vi "AI Read with state .vi"(0 "taskID in":u32 format="%x", 1 "conditional retrieval (off)":T2={"mode (off)"=enum."off", "channel index (0)"=0, "slope (rising)"=enum."rising", "level (0.0)"=0.0, "hysteresis (0.0)"=0.0, "skip count (0)"=0, "offset (0)"=0} {"hysteresis (0.0)" format="%0.2f"; "level (0.0)" format="%0.2f"}, 5 "number of scans to read (-1:all)":i32=-1, 7 "time limit in sec (-1:auto calculate)":sgl=-1.0 format="%0.2f", 11 "error in (no error)":errorcluster, 12 "read/search position (from mark)":T3={"position (rel. to mark:1)"=enum."relative to read mark", "read offset (0)"=0}) -> (2 "scan backlog":u32, 3 "number read":i32, 4 "taskID out":u32 format="%x", 6 "scaled data":sgl[][](array[numeric]) format="%0.6f", 10 "retrieval complete":bool, 14 "acquisition state":T1(ring)=enum."no acquisition", 15 "error out":errorcluster)   [LabVIEW 2019]
doc: "Reads data from a buffered data acquisition."
uses:
  AI Buffer Read (scaled array).vi
panel:
  # "scan #"
  # "channel"
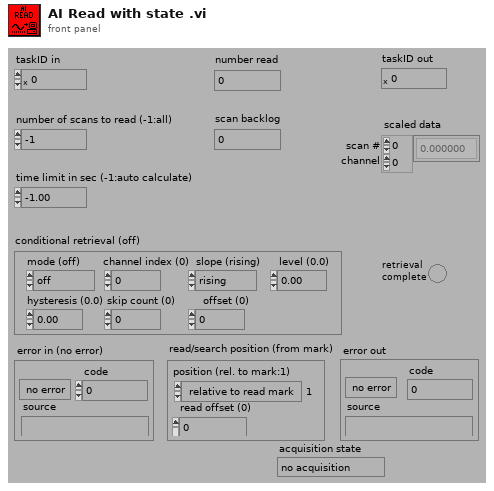
[diagram p1: front panel]
types:
  T1 = enum16{"running", "finished w/ backlog", "finished w/o backlog", "paused", "no acquisition"}
  T2 = cluster{"mode (off)":enum16{"no change", "off", "on"}, "channel index (0)":i32, "slope (rising)":enum16{"no change", "rising", "falling"}, "level (0.0)":sgl, "hysteresis (0.0)":sgl, "skip count (0)":i32, "offset (0)":i32}
  T3 = cluster{"position (rel. to mark:1)":enum16{"no change", "relative to read mark", "relative to start of buffer", "relative to end of data", "relative to trigger point"}, "read offset (0)":i32}
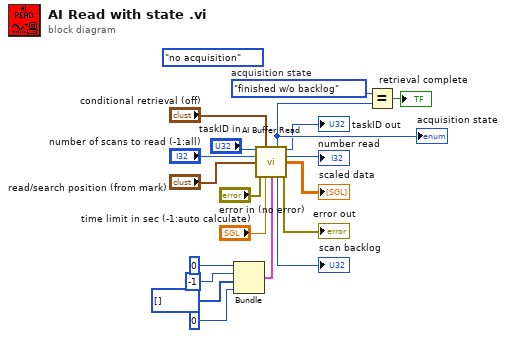
[diagram p0: block diagram]
diagram:
  (unwired) T1."no acquisition" ("acquisition state")
  w4 = T1."finished w/o backlog"  # acquisition state
  n1 = Bundle(u16 0, -1, i32[] [], u32 0) -> (w10:cluster{u16, i32, i32[], u32})  [unwired: 1 in]
  n2 = call-poly "AI Buffer Read.vi"("task ID"="taskID in", "conditional retrieval specification (off)"="conditional retrieval (off)", "number to read (-1: no change)"="number of scans to read (-1:all)", "read/search location (no change)"="read/search position (from mark)", "error in (no error)"="error in (no error)", "time limit (-1: auto calculate)"="time limit in sec (-1:auto calculate)", "read specification (no change)"=w10) -> ("acquisition state"=w15:T1, "task ID out"=→"taskID out":u32, "number read"=→"number read":i32, "scaled data"=→"scaled data":sgl[][], "scan backlog"=→"scan backlog":u32, "error out"=→"error out":errorcluster)  [unwired: 2 in, 1 out]
  "acquisition state" <- w15
  n3 = Equal?(x=w4, y=w15) -> (x = y?=→"retrieval complete":bool)
